vi "ex7-5.vi"   [LabVIEW 2013]
uses:
  <vilib>/NXT/Block Support/NXT_InputPort.ctl
  <vilib>/NXT/Block Support/NXT_OutputPort.ctl
  <vilib>/NXT/Dual Mode Library/Sensors/Touch_Pressed.vi
  <vilib>/NXT/NXTIO Xnodes/NXTIONodeSubVIs/NXTStopMotors.vi
  <vilib>/NXT/NXTIO Xnodes/NXTIONodeSubVIs/NXTMoveMotors.vi
  <vilib>/NXT/Subs/LVHSConnector.ctl
  <vilib>/NXT/NXTIO Xnodes/AddressXNode/NXTIOAddress.xnode
  <vilib>/NXT/NXTIO Xnodes/NXTIOXNode/NXTIO.xnode
  <vilib>/NXT/LegoClasses/BrickReference/BrickReference.lvclass
types:
  T1 = typedef "NXT_InputPort.ctl" = u32
  T2 = typedef "NXT_OutputPort.ctl" = u8
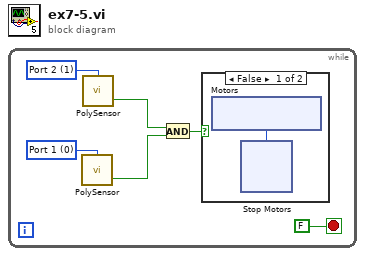
[diagram p0: block diagram]
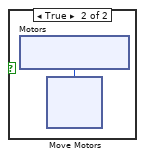
[diagram p2: hidden frame]
diagram:
  n1 = while {
    stop <- FALSE stop-if-true
    w2 = T1 0 items=["Port 1", "Port 2", "Port 3", "Port 4"] ("Port (Port 1)")
    w3 = T1 1 items=["Port 1", "Port 2", "Port 3", "Port 4"] ("Port (Port 1)")
    n2 = call-poly <vilib>:"PolySensor.vi"("Port (Port 1)"=w2) -> ("Yes / No"=w4:bool)  [unwired: 2 in, 1 out]
    n3 = call-poly <vilib>:"PolySensor.vi"("Port (Port 1)"=w3) -> ("Yes / No"=w5:bool)  [unwired: 2 in, 1 out]
    n4 = And(x=w5, y=w4) -> (x .and. y?=w6:bool)
    n5 = case shown="False" w6 {
      frame False {
        n6 = xnode "Motors"() -> ("Motor"=w7:T2)
        n7 = xnode "Stop Motors"("Motors"=w7) -> ()  [unwired: 1 in, 1 out]
      }
      frame True {
        n8 = xnode "Motors"() -> ("Motor"=w14:T2)
        n9 = xnode "Move Motors"("Motors"=w14) -> ()  [unwired: 2 in, 1 out]
      }
    }
  }
